vi "Scan API List.vi"(8 "error in (no error)":errorcluster, 10 "SMO":refnum<class "SMO.lvclass">) -> (0 "error out":errorcluster, 2 "Public API":T1(array[cluster]))   [LabVIEW 2013, in "Registry-SMO.lvclass"]
uses:
  Registry-SMO.lvclass
  SMO/SMO.lvclass
  <vilib>/Utility/VariantDataType/Type.ctl
  <vilib>/Utility/VariantDataType/VariantType.lvlib
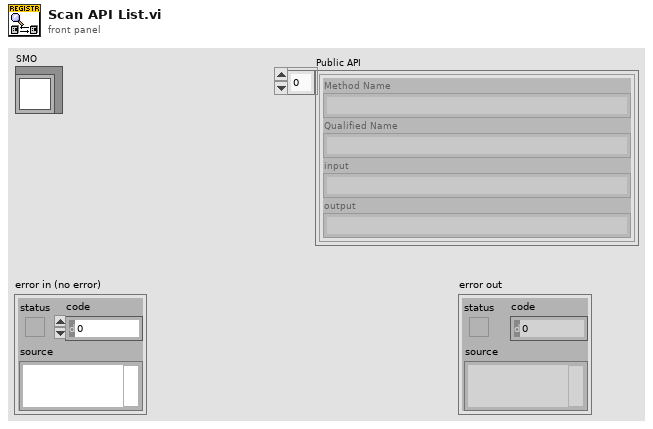
[diagram p1: front panel]
types:
  T1 = cluster{"Method Name":string, "Qualified Name":string, "input":string, "output":string}[]
  T2 = enum32{"invalid scope", "public", "private", "protected", "community"}
  T3 = typedef "VariantType.lvlib/Type.ctl" = enum8{"Invalid Type", "Void", "I8", "I16", "I32", "I64", "U8", "U16", "U32", "U64", "Single Float", "Double Float", "Extended Float", "Single Complex", "Double Complex", "Extended Complex", "Enum U8", "Enum U16", "Enum U32", "Enum U64", "Single Float With Unit", "Double Float With Unit", "Extended Float With Unit", "Single Complex with Unit", "Double Complex with Unit", "Extended Complex with Unit", "Boolean", "String", "Path", "Picture", "Tag", "Array", "Cluster", "Variant", "LV Variant", "Waveform", "Timestamp", "Digital Waveform", "Digital Data", "ExpressData", "Refnum", "External Data", "VI", "Poly VI", "LabVIEW Class Instance", "Fixed Point"}
  T4 = cluster{string, string, string, "trimmed string":string}
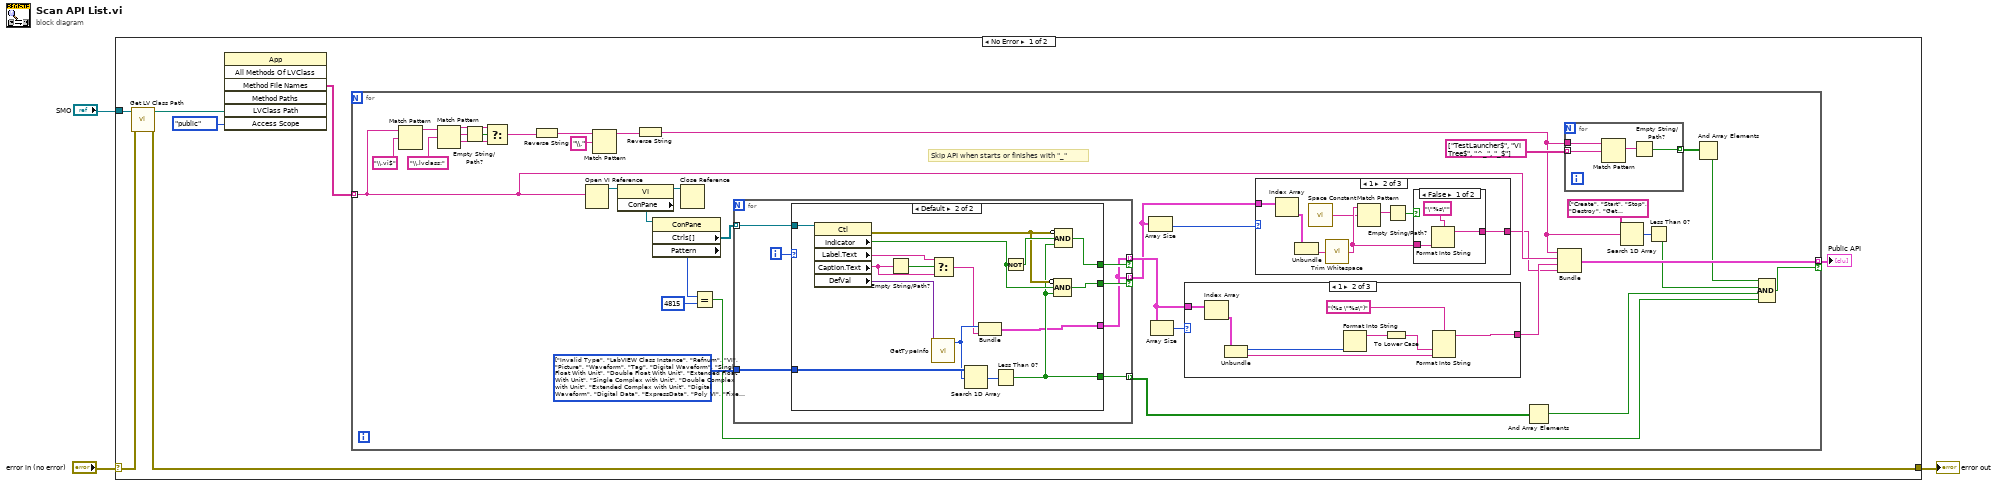
[diagram p0: block diagram]
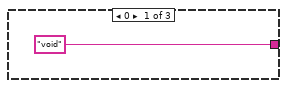
[diagram p2: hidden frame]
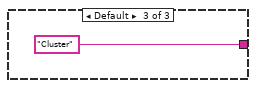
[diagram p4: hidden frame]
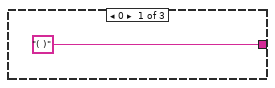
[diagram p5: hidden frame]
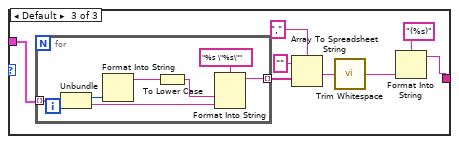
[diagram p6: hidden frame]
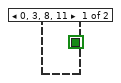
[diagram p7: hidden frame]
diagram:
  n1 = case shown="No Error" "error in (no error)" {
    selector: "error in (no error)" -> [w7 w114]
    tunnel: [w6 w114] -> w2
    tunnel: "SMO" -> [w10 _]
    frame No Error {
      n2 = call <vilib>:"Get LV Class Path.vi"("error in (no error)"=w7, "object"=w10) -> ("error out"=w6:errorcluster, "class path"=w9:path)  [unwired: 8 in]
      n3 = invoke class="App" method="All Methods Of LVClass"("LVClass Path"=w9, "Access Scope"=T2."public") -> ("Method File Names"=w5:string[])  [unwired: 5 in, 6 out]
      n4 = for {
        tunnel: w5 -> [w35] mode=indexing
        tunnel: [w45] -> w4 mode=indexing if=w29
        w34 = T3[] [enum."Invalid Type", enum."LabVIEW Class Instance", enum."Refnum", enum."VI", enum."Picture", enum."Waveform", enum."Tag", enum."Digital Waveform", enum."Single Float With Unit", enum."Double Float With Unit", enum."Extended Float With Unit", enum."Single Complex with Unit", enum."Double Complex with Unit", enum."Extended Complex with Unit", enum."Digital Waveform", enum."Digital Data", enum."ExpressData", enum."Poly VI", enum."Fixed Point"] items=["Invalid Type", "Void", "I8", "I16", "I32", "I64", "U8", "U16", "U32", "U64", "Single Float", "Double Float", "Extended Float", "Single Complex", "Double Complex", "Extended Complex", "Enum U8", "Enum U16", "Enum U32", "Enum U64", "Single Float With Unit", "Double Float With Unit", "Extended Float With Unit", "Single Complex with Unit", "Double Complex with Unit", "Extended Complex with Unit", "Boolean", "String", "Path", "Picture", "Tag", "Array", "Cluster", "Variant", "LV Variant", "Waveform", "Timestamp", "Digital Waveform", "Digital Data", "ExpressData", "Refnum", "External Data", "VI", "Poly VI", "LabVIEW Class Instance", "Fixed Point"]
        # "Skip API when starts or finishes with \"_\""
        n5 = Match Pattern(string=w35, regular expression="\\.vi$") -> (before substring=w37:string)  [unwired: 1 in, 3 out]
        n6 = Match Pattern(string=w37, regular expression="\\.lvclass:") -> (before substring=w41:string, match substring=w39:string, after substring=w42:string)  [unwired: 1 in, 1 out]
        n7 = Empty String/Path?(string/path=w39) -> (empty?=w40:bool)
        n8 = Select(t=w41, s=w40, f=w42) -> (s? t:f=w22:string)
        n9 = Reverse String(1:w22) -> (0:w25:string)
        n10 = Open VI Reference(vi path=w35) -> (vi reference=w47:refnum<vi>)  [unwired: 5 in, 1 out]
        n11 = Match Pattern(string=w25, regular expression="\\.") -> (before substring=w23:string)  [unwired: 1 in, 3 out]
        n12 = property class="VI"(reference=w47) -> (reference out=w46:refnum<vi>, "ConPane"=w44:refnum<vi>)  [unwired: 1 in, 1 out]
        n13 = Reverse String(1:w23) -> (0:w21:string)
        n14 = property class="ConPane"(reference=w44) -> ("Ctrls[]"=w43:refnum<vi>[], "Pattern"=w20:u32)  [unwired: 1 in, 2 out]
        n15 = Close Reference(reference=w46) -> ()  [unwired: 1 in, 1 out]
        n16 = Equal?(x=w20, y=u32 4815) -> (x = y?=w18:bool)
        n17 = for {
          tunnel: w43 -> [w94] mode=indexing
          tunnel: [w90] -> w15 mode=indexing if=w96
          tunnel: [w90] -> w11 mode=indexing if=w95
          tunnel: w34 -> [w92]
          tunnel: [w91] -> w16 mode=indexing
          i -> [w93]
          n18 = case shown="Default" w93 {
            tunnel: [_ w112] -> w96
            tunnel: [_ w109] -> w95
            tunnel: [_ w98] -> w90
            tunnel: w94 -> [_ w108]
            tunnel: w92 -> [_ w106]
            tunnel: [TRUE w104] -> w91
            frame 0, 3, 8, 11 {
            }
            frame Default {
              n19 = property class="Ctl"(reference=w108) -> (error out=w111:errorcluster, "Indicator"=w110:bool, "Label.Text"=w101:string, "Caption.Text"=w102:string, "DefVal"=w107:variant)  [unwired: 1 in, 1 out]
              n20 = Empty String/Path?(string/path=w102) -> (empty?=w103:bool)
              n21 = call <vilib>:"GetTypeInfo.vi"("Variant"=w107) -> ("Type Enum"=w100:T3)  [unwired: 6 in, 4 out]
              n22 = Select(t=w101, s=w103, f=w102) -> (s? t:f=w99:string)
              n23 = Search 1D Array(1D array=w106, element=w100) -> (index of element=w105:i32)  [unwired: 1 in]
              n24 = Bundle("Type Enum"=w100, "Caption.Text"=w99) -> (w98:cluster{"Type Enum":T3, "Caption.Text":string})  [unwired: 1 in]
              n25 = Less Than 0?(x=w105) -> (x < 0?=w104:bool)
              n26 = Not(x=w110) -> (.not. x?=w113:bool)
              n27 = Compound Arithmetic op=AND(invert w111, w110, w104) -> (w109:bool)
              n28 = Compound Arithmetic op=AND(invert w111, w113, w104) -> (w112:bool)
            }
          }
        }
        n29 = Array Size(array=w11) -> (size(s)=w12:i32)
        n30 = Array Size(array=w15) -> (size(s)=w17:i32)
        n31 = case shown="1" w17 {
          tunnel: w15 -> [_ w70 w78]
          tunnel: ["( )" w66 w75] -> w14
          frame 0 {
          }
          frame 1 {
            n32 = Index Array(array=w70) -> (element=w68:cluster{"Type Enum":T3, "Caption.Text":string})  [unwired: 1 in]
            n33 = Unbundle(w68) -> ("Type Enum"=w65:T3, "Caption.Text"=w67:string)
            n34 = Format Into String(w65) -> (resulting string=w64:string)  [unwired: 3 in, 1 out]
            n35 = To Lower Case(string=w64) -> (all lower case string=w63:string)
            n36 = Format Into String(format string="(%s \"%s\")", w63, w67) -> (resulting string=w66:string)  [unwired: 2 in, 1 out]
          }
          frame Default {
            n37 = for {
              tunnel: [w83] -> w77 mode=indexing
              tunnel: w78 -> [w82] mode=indexing
              n38 = Unbundle(w82) -> ("Type Enum"=w80:T3, "Caption.Text"=w84:string)
              n39 = Format Into String(w80) -> (resulting string=w81:string)  [unwired: 3 in, 1 out]
              n40 = To Lower Case(string=w81) -> (all lower case string=w79:string)
              n41 = Format Into String(format string="%s \"%s\"", w79, w84) -> (resulting string=w83:string)  [unwired: 2 in, 1 out]
            }
            n42 = Array To Spreadsheet String(delimiter (Tab)=",", array=w77, 3:"" ("format string")) -> (spreadsheet string=w76:string)
            n43 = call <vilib>:"Trim Whitespace.vi"("string"=w76) -> ("trimmed string"=w71:string)  [unwired: 1 in]
            n44 = Format Into String(format string="(%s)", w71) -> (resulting string=w75:string)  [unwired: 2 in, 1 out]
          }
        }
        n45 = case shown="1" w12 {
          tunnel: w11 -> [_ w56 _]
          tunnel: ["void" w54 "Cluster"] -> w13
          frame 0 {
          }
          frame 1 {
            n46 = Index Array(array=w56) -> (element=w55:cluster{"Type Enum":T3, "Caption.Text":string})  [unwired: 1 in]
            n47 = Unbundle(w55) -> ("Caption.Text"=w53:string)  [unwired: 1 out]
            n48 = call <vilib>:"Space Constant.vi"() -> ("String"=w51:string)
            n49 = call <vilib>:"Trim Whitespace.vi"("string"=w53) -> ("trimmed string"=w52:string)  [unwired: 1 in]
            n50 = Match Pattern(string=w52, regular expression=w51) -> (match substring=w50:string)  [unwired: 1 in, 3 out]
            n51 = Empty String/Path?(string/path=w50) -> (empty?=w49:bool)
            n52 = case shown="False" w49 {
              tunnel: [w58 w60] -> w54
              tunnel: w52 -> [w57 w60]
              frame False {
                n53 = Format Into String(format string="\"%s\"", w57) -> (resulting string=w58:string)  [unwired: 2 in, 1 out]
              }
              frame True {
              }
            }
          }
          frame Default {
          }
        }
        n54 = And Array Elements(Boolean array=w16) -> (logical AND=w30:bool)
        n55 = Bundle(w21, w35, w14, "trimmed string"=w13) -> (w45:T4)  [unwired: 1 in]
        n56 = for {
          tunnel: w21 -> [w89]
          tunnel: string[] ["TestLauncher$", "VI Tree$", "^_", "_$"] -> [w88] mode=indexing
          tunnel: [w86] -> w27 mode=indexing
          n57 = Match Pattern(string=w89, regular expression=w88) -> (match substring=w87:string)  [unwired: 1 in, 3 out]
          n58 = Empty String/Path?(string/path=w87) -> (empty?=w86:bool)
        }
        n59 = Search 1D Array(1D array=string[] ["Create", "Start", "Stop", "Destroy", "Get PublicEventRegistration"], element=w21) -> (index of element=w32:i32)  [unwired: 1 in]
        n60 = Less Than 0?(x=w32) -> (x < 0?=w31:bool)
        n61 = And Array Elements(Boolean array=w27) -> (logical AND=w26:bool)
        n62 = Compound Arithmetic op=AND(w26, w31, w30, w18) -> (w29:bool)
      }
      "Public API" <- w4
    }
    frame Error {
    }
  }
  "error out" <- w2
